vi "UpdateMeasurementDirectory.vi"(8 "error in (no error)":errorcluster, 10 "Measurement Directory":path, 11 "ViewerManager in":refnum<class "ViewerManager.lvclass">) -> (0 "error out":errorcluster, 3 "ViewerManager out":refnum<class "ViewerManager.lvclass">)   [LabVIEW 2019, in "ViewerManager.lvlib" / "ViewerManager.lvclass"]
uses:
  ViewerManager.lvclass
  ViewerManager.lvclass/ViewerManager.ctl
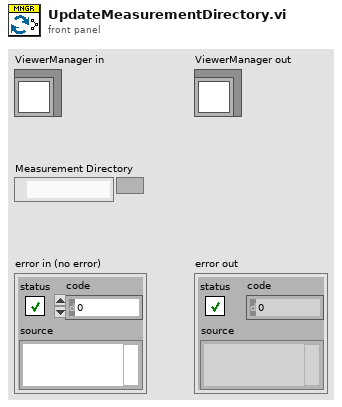
[diagram p1: front panel]
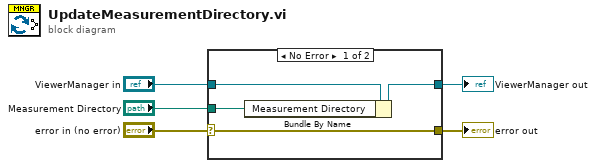
[diagram p0: block diagram]
diagram:
  n1 = case shown="No Error" "error in (no error)" {
    selector: "error in (no error)" -> [w9 w11]
    tunnel: [w9 w11] -> w4
    tunnel: [w7 w10] -> w2
    tunnel: "ViewerManager in" -> [w8 w10]
    tunnel: "Measurement Directory" -> [w6 _]
    frame No Error {
      n2 = Bundle By Name(cluster=w8, "Measurement Directory"=w6) -> (w7:refnum<class "ViewerManager.lvclass">)
    }
    frame Error {
    }
  }
  "error out" <- w4
  "ViewerManager out" <- w2
